vi "CheckMasterConnection.vi"(3 "Master IP":string="Master IP") -> (0 "error out":errorcluster, 1 "Master There?":bool)   [LabVIEW 2014]
doc: "Returns true if it was able to open a connection to the ROS Master"
uses:
  <userlib>/ROS for LabVIEW Software.lnk/ROS/Code/_ROSDefinition.vi
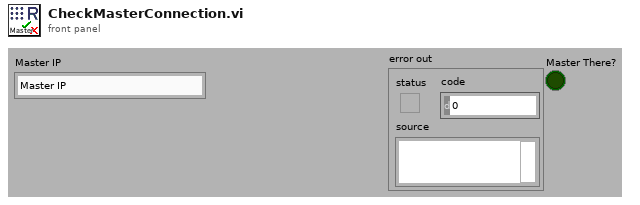
[diagram p1: front panel]
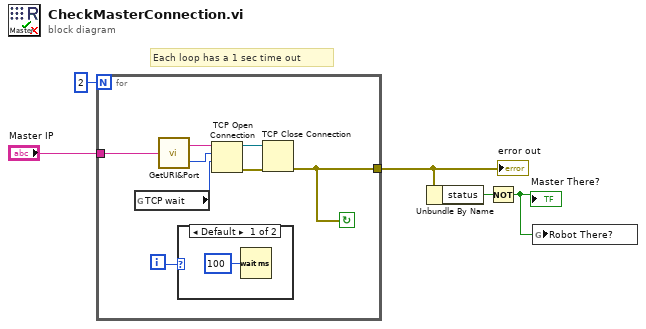
[diagram p0: block diagram]
diagram:
  # "Each loop has a 1 sec time out"
  n1 = for {
    N: 2 -> [_]
    tunnel: "Master IP" -> [w13]
    tunnel: [w7] -> w4
    i -> [w6]
    stop <- w7 continue-if-true
    n2 = global read "_ROSDefinition.vi" "TCP wait"() -> (w8:i32)
    n3 = call <userlib>:"GetURI&Port.vi"("URI in"=w13) -> ("Port"=w11:u16, "URI"=w12:string)
    n4 = case shown="Default" w6 {
      frame Default {
        n5 = Wait (ms)(milliseconds to wait=u32 100) -> ()  [unwired: 1 out]
      }
      frame 0 {
      }
    }
    n6 = TCP Open Connection(address=w12, remote port or service name=w11, timeout ms (60000)=w8) -> (connection ID=w9:refnum<k5>, error out=w10:errorcluster)  [unwired: 2 in]
    n7 = TCP Close Connection(connection ID=w9, error in (no error)=w10) -> (error out=w7:errorcluster)  [unwired: 1 in, 1 out]
  }
  "error out" <- w4
  n8 = Unbundle By Name(w4) -> ("status"=w3:bool)
  n9 = Not(x=w3) -> (.not. x?=w2:bool)
  "Master There?" <- w2
  n10 = global write "_ROSDefinition.vi" "Robot There?"(w2) -> ()
